vi "Determine Device Types.vi"(10 "DeviceIDs":T1[](array[typedef])) -> (3 "Device Classes":string[](array[string]))   [LabVIEW 2018]
doc: "This VI returns the device types (e.g., PCC, Smart Relay, PV) for the associated device IDs."
uses:
  <vilib>/ORNL/CSEISMIC DDS/CSEISMIC DDS Base/Data Types/Controls/DeviceClass Selector.ctl
  <vilib>/ORNL/CSEISMIC DDS/CSEISMIC DDS Base/Data Types/Controls/DeviceID.ctl
  <vilib>/ORNL/CSEISMIC DDS/CSEISMIC DDS Base/CSEISMIC DDS.lvclass
panel:
  out "Device Type":T2 format="%04x" items=["Invalid"=0, "IED"=256, "DER"=512, "Relay"=768, "Meter"=1024, "Load"=1280, "Forecast"=1536, "Price"=1792, "Energy Storage"=513, "PV"=514, "Generator"=515, "Smart Relay"=769, "PCC"=770, "Smart Meter"=1025, "PMU"=1026, "HVAC"=1281]
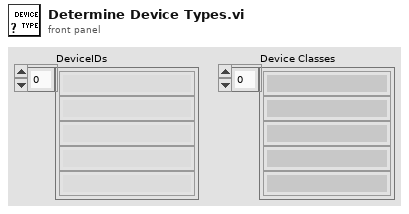
[diagram p1: front panel]
types:
  T1 = typedef "CSEISMIC DDS.lvlib/CSEISMIC DDS.lvclass/DeviceID.ctl" = string
  T2 = typedef "CSEISMIC DDS.lvlib/CSEISMIC DDS.lvclass/DeviceClass Selector.ctl" = u16
  T3 = typedef "LVStringsAndValuesArrayTypeDef_U16.ctl" = cluster{"String":string, "Value":u16}[]
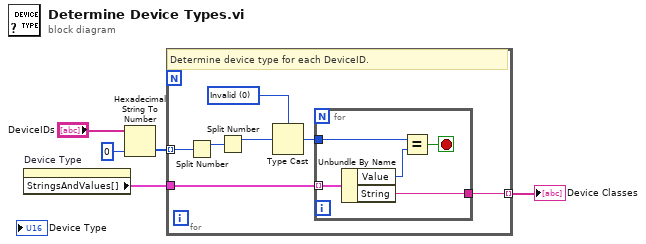
[diagram p0: block diagram]
diagram:
  n1 = property on="Device Type" class="Ring (strict)"() -> ("StringsAndValues[]"=w4:T3)  [unwired: 2 in, 2 out]
  n2 = Hexadecimal String To Number(string="DeviceIDs", default (0uL)=u64 0 ("default (0 U32)")) -> (number=w2:u64[])  [unwired: 1 in, 1 out]
  n3 = for {
    tunnel: w2 -> [w11] mode=indexing
    tunnel: w4 -> [w9]
    tunnel: [w7] -> w5 mode=indexing
    w8 = T2 0 items=["Invalid"=0, "IED"=256, "DER"=512, "Relay"=768, "Meter"=1024, "Load"=1280, "Forecast"=1536, "Price"=1792, "Energy Storage"=513, "PV"=514, "Generator"=515, "Smart Relay"=769, "PCC"=770, "Smart Meter"=1025, "PMU"=1026, "HVAC"=1281] ("*(type *) &x 4")
    # "Determine device type for each DeviceID."
    n4 = Split Number(x=w11) -> (hi(x)=w12:u32)  [unwired: 1 out]
    n5 = Split Number(x=w12) -> (hi(x)=w10:u16)  [unwired: 1 out]
    n6 = Type Cast(type=w8, x=w10) -> (*(type *) &x=w6:T2)
    n7 = for {
      tunnel: w9 -> [w14] mode=indexing
      tunnel: w6 -> [w15]
      tunnel: [w13] -> w7
      stop <- w17 stop-if-true
      n8 = Unbundle By Name(w14) -> ("Value"=w16:u16, "String"=w13:string)
      n9 = Equal?(x=w15, y=w16) -> (x = y?=w17:bool)
    }
  }
  "Device Classes" <- w5
